vi "NI VeriStand - Move Custom Device Item.vi"(7 "Highlight? (F)":bool, 8 "error in (no error)":errorcluster, 10 "New Parent Ref in":T1 format="%.0x", 11 "Item Ref in":T1 format="%.0x") -> (0 "error out":errorcluster, 3 "Item Ref out":T1 format="%.0x", 4 "Moved?":bool)   [LabVIEW 2020, in "Custom Device Offline API.lvlib"]
uses:
  <vilib>/NI VeriStand/Custom Device Offline API/Custom Device Offline API.lvlib
  <vilib>/NI VeriStand/Custom Device API/Custom Device Item Ref.ctl
  NationalInstruments.VeriStand.SystemDefinitionAPI
  <vilib>/NI VeriStand/Custom Device API/Custom Device API.lvlib
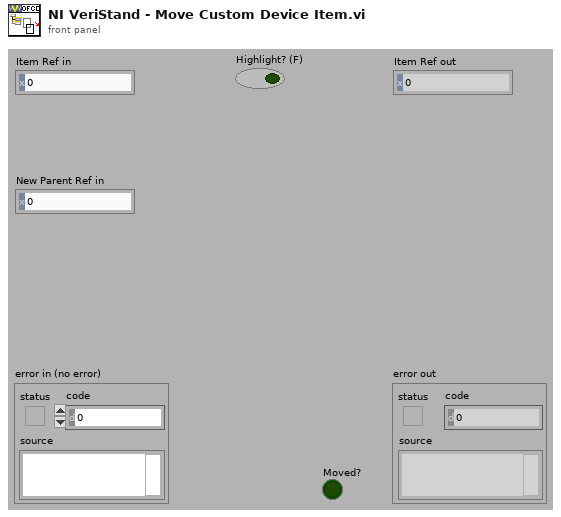
[diagram p1: front panel]
types:
  T1 = typedef "Custom Device API.lvlib/Custom Device Item Ref.ctl" = u64
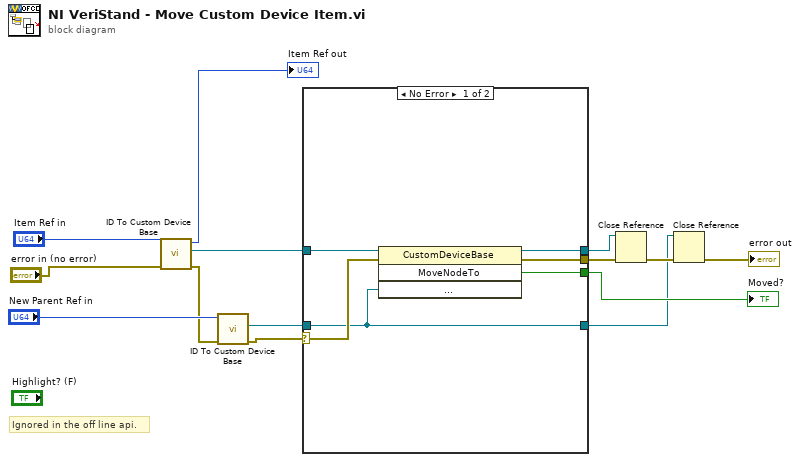
[diagram p0: block diagram]
diagram:
  # "Ignored in the off line api."
  n1 = call <vilib>:"ID To Custom Device Base.vi"("error in (no error)"="error in (no error)", "ID in"="Item Ref in") -> ("error out"=w11:errorcluster, "BaseNode"=w9:refnum<k24>, "ID out"=→"Item Ref out":u64)  [unwired: 7 in]
  n2 = call <vilib>:"ID To Custom Device Base.vi"("error in (no error)"=w11, "ID in"="New Parent Ref in") -> ("error out"=w10:errorcluster, "BaseNode"=w8:refnum<k24>)  [unwired: 7 in, 1 out]
  n3 = case shown="No Error" w10 {
    selector: w10 -> [w19 w23]
    tunnel: w9 -> [w20 w22]
    tunnel: w8 -> [w15 w21]
    tunnel: [w18 _] -> w7
    tunnel: [w17 w23] -> w5
    tunnel: [w16 w22] -> w2
    tunnel: [w15 w21] -> w1
    frame No Error {
      n4 = invoke class="CustomDeviceBase" method="MoveNodeTo"(reference=w20, error in=w19, "ParentType"=w15) -> (reference out=w16:refnum<k24>, error out=w17:errorcluster, "MoveNodeTo"=w18:bool)  [unwired: 1 in, 1 out]
    }
    frame Error {
    }
  }
  "Moved?" <- w7
  n5 = Close Reference(reference=w2, error in (no error)=w5) -> (error out=w3:errorcluster)
  n6 = Close Reference(reference=w1, error in (no error)=w3) -> (error out=→"error out":errorcluster)
